vi "Auto Execute Commands.vi"(11 "Auto Commands":T1=[{"Drive Duration"=0.0, "Left Speed"=0.0, "Right Speed"=0.0, "Set Point"=1.0, "Set Point Duration"=2.0, "Command"=enum."Shooter", "Wait ms"=0.0, "Recorded Filename"=enum."pickup2balls"}]) -> ()   [LabVIEW 2019]
uses:
  <vilib>/Rock Robotics/WPI/Solenoid/WPI_SolenoidValue.ctl
  <vilib>/Rock Robotics/WPI/Solenoid/WPI_SolenoidSetEnum.vi
  Controls/Auto Controls.ctl
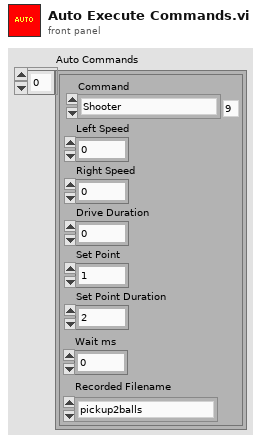
[diagram p1: front panel]
types:
  T1 = typedef "Auto Controls.ctl" = cluster{"Drive Duration":dbl, "Left Speed":dbl, "Right Speed":dbl, "Set Point":dbl, "Set Point Duration":dbl, "Command":enum16{"", "Drive Forwards", "Drive Backwards", "Stop", "Turn Left", "Turn Right", "Drop Intake", "Lift Intake", "Intake", "Shooter", "Transfer", "Wait", "Drive from recorded file"}, "Wait ms":dbl, "Recorded Filename":enum16{"pickup2balls", "drivetoshoot", "pickup5balls", "drivetoshoot5balls"}}[]
  T2 = typedef "WPI_SolenoidValue.ctl" = enum16{"Off", "On", "Forward", "Reverse"}
  T3 = enum16{"", "Drive Forwards", "Drive Backwards", "Stop", "Turn Left", "Turn Right", "Drop Intake", "Lift Intake", "Intake", "Shooter", "Transfer", "Wait", "Drive from recorded file"}
  T4 = enum16{"pickup2balls", "drivetoshoot", "pickup5balls", "drivetoshoot5balls"}
  T5 = typedef "WPI_SolenoidDevRef.ctl" = cluster{"DevStatus":errorcluster, "Pneumatics Control Module":u8, "Forward Solenoid Channel":T6, "Reverse Solenoid Channel":T6}
  T6 = typedef "WPI_SolenoidChannel.ctl" = enum8{"Solenoid 0", "Solenoid 1", "Solenoid 2", "Solenoid 3", "Solenoid 4", "Solenoid 5", "Solenoid 6", "Solenoid 7", "Invalid"}
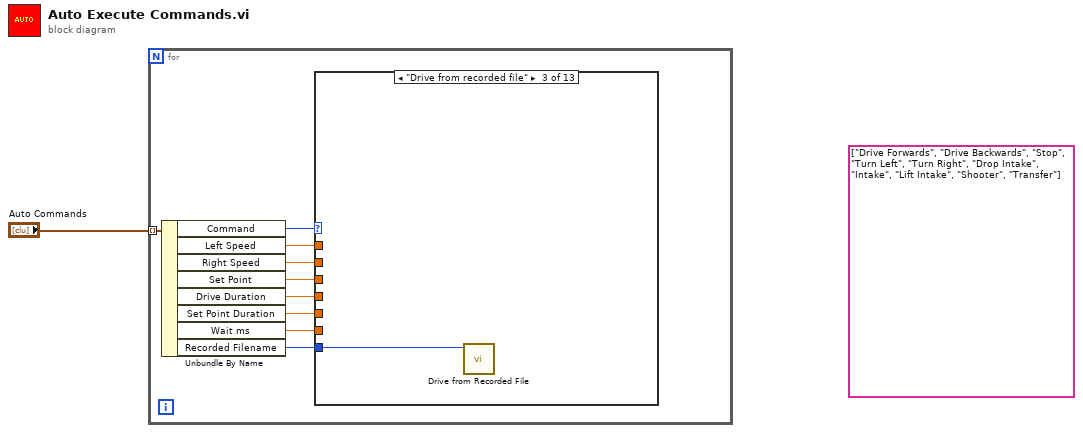
[diagram p0: block diagram]
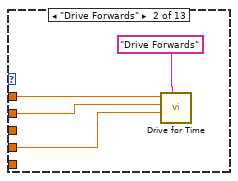
[diagram p3: hidden frame]
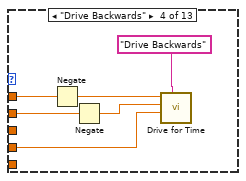
[diagram p4: hidden frame]
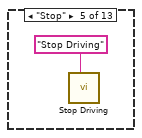
[diagram p5: hidden frame]
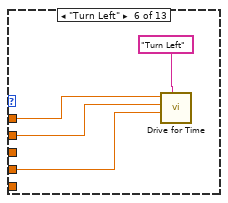
[diagram p6: hidden frame]
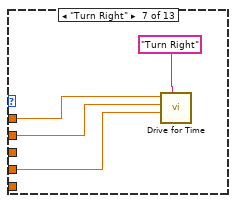
[diagram p7: hidden frame]
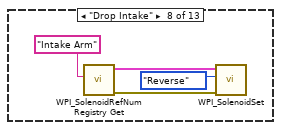
[diagram p8: hidden frame]
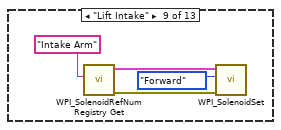
[diagram p9: hidden frame]
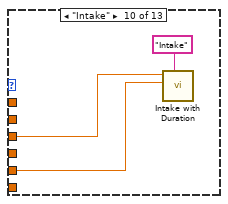
[diagram p10: hidden frame]
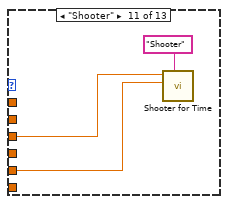
[diagram p11: hidden frame]
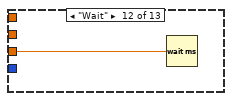
[diagram p12: hidden frame]
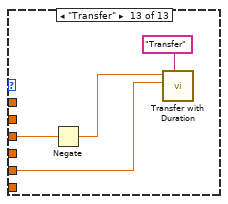
[diagram p13: hidden frame]
diagram:
  (unwired) string[] ["Drive Forwards", "Drive Backwards", "Stop", "Turn Left", "Turn Right", "Drop Intake", "Intake", "Lift Intake", "Shooter", "Transfer"]
  n1 = for {
    tunnel: "Auto Commands" -> [w10] mode=indexing
    n2 = Unbundle By Name(w10) -> ("Command"=w9:T3, "Left Speed"=w8:dbl, "Right Speed"=w7:dbl, "Set Point"=w5:dbl, "Drive Duration"=w6:dbl, "Set Point Duration"=w4:dbl, "Wait ms"=w3:dbl, "Recorded Filename"=w2:T4)
    n3 = case shown="\"Drive from recorded file\"" w9 {
      tunnel: w8 -> [_ w13 _ w20 _ w25 w29 _ _ _ _ _ _]
      tunnel: w7 -> [_ w12 _ w19 _ w24 w28 _ _ _ _ _ _]
      tunnel: w6 -> [_ w11 _ w18 _ w23 w27 _ _ _ _ _ _]
      tunnel: w5 -> [_ _ _ _ _ _ _ _ _ w40 w43 _ w48]
      tunnel: w4 -> [_ _ _ _ _ _ _ _ _ w39 w42 _ w46]
      tunnel: w3 -> [_ _ _ _ _ _ _ _ _ _ _ w45 _]
      tunnel: w2 -> [_ _ w15 _ _ _ _ _ _ _ _ _ _]
      frame Default {
      }
      frame "Drive Forwards" {
        n4 = call "Drive for Time.vi"("Description"="Drive Forwards", "Seconds"=w11, "Right Speed"=w12, "Left Speed"=w13) -> ()  [unwired: 7 in, 1 out]
      }
      frame "Drive from recorded file" {
        n5 = call "Drive from Recorded File.vi"("Recorded Filename"=w15) -> ()  [unwired: 11 in]
      }
      frame "Drive Backwards" {
        n6 = Negate(x=w20) -> (-x=w17:dbl)
        n7 = Negate(x=w19) -> (-x=w16:dbl)
        n8 = call "Drive for Time.vi"("Description"="Drive Backwards", "Seconds"=w18, "Right Speed"=w16, "Left Speed"=w17) -> ()  [unwired: 7 in, 1 out]
      }
      frame "Stop" {
        n9 = call "Stop Driving.vi"("Description"="Stop Driving") -> ()  [unwired: 10 in, 1 out]
      }
      frame "Turn Left" {
        n10 = call "Drive for Time.vi"("Description"="Turn Left", "Seconds"=w23, "Right Speed"=w24, "Left Speed"=w25) -> ()  [unwired: 7 in, 1 out]
      }
      frame "Turn Right" {
        n11 = call "Drive for Time.vi"("Description"="Turn Right", "Seconds"=w27, "Right Speed"=w28, "Left Speed"=w29) -> ()  [unwired: 7 in, 1 out]
      }
      frame "Drop Intake" {
        n12 = call <vilib>:"WPI_SolenoidRefNum Registry Get.vi"("refnum name"="Intake Arm") -> ("error out"=w32:errorcluster, "SolenoidDevRef"=w33:T5)  [unwired: 9 in]
        n13 = call-poly <vilib>:"WPI_SolenoidSet.vi"("error in (no error)"=w32, "Value"=WPI_SolenoidValue."Reverse", "SolenoidDevRef"=w33) -> ()  [unwired: 7 in, 2 out]
      }
      frame "Lift Intake" {
        n14 = call <vilib>:"WPI_SolenoidRefNum Registry Get.vi"("refnum name"="Intake Arm") -> ("error out"=w36:errorcluster, "SolenoidDevRef"=w37:T5)  [unwired: 9 in]
        n15 = call-poly <vilib>:"WPI_SolenoidSet.vi"("error in (no error)"=w36, "Value"=WPI_SolenoidValue."Forward", "SolenoidDevRef"=w37) -> ()  [unwired: 7 in, 2 out]
      }
      frame "Intake" {
        n16 = call "Intake with Duration.vi"("Description"="Intake", "Duration (s)"=w39, "Setpoint"=w40) -> ()  [unwired: 8 in, 1 out]
      }
      frame "Shooter" {
        n17 = call "Shooter for Time.vi"("Description"="Shooter", "Duration (s)"=w42, "Setpoint"=w43) -> ()  [unwired: 8 in, 1 out]
      }
      frame "Wait" {
        n18 = Wait (ms)(milliseconds to wait=w45) -> ()  [unwired: 1 out]
      }
      frame "Transfer" {
        n19 = Negate(x=w48) -> (-x=w47:dbl)
        n20 = call "Transfer with Duration.vi"("Description"="Transfer", "Duration (s)"=w46, "Setpoint"=w47) -> ()  [unwired: 8 in, 1 out]
      }
    }
  }
